vi "Write Data.vi"(8 "error in":errorcluster, 10 "Data":u16, 11 "U16 in":refnum<class "U16.lvclass">) -> (0 "error out":errorcluster, 3 "U16 out":refnum<class "U16.lvclass">)   [LabVIEW 2012, in "Base Data Class.lvlib" / "U16.lvclass"]
uses:
  U16.lvclass
  U16.lvclass/U16.ctl
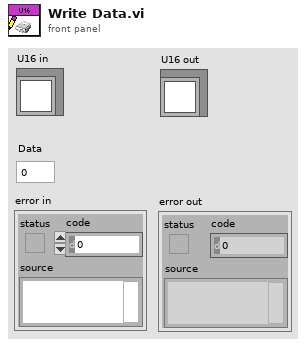
[diagram p1: front panel]
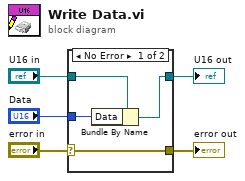
[diagram p0: block diagram]
diagram:
  n1 = case shown="No Error" "error in" {
    selector: "error in" -> [w9 w10]
    tunnel: [w9 w10] -> w4
    tunnel: [w7 w11] -> w2
    tunnel: "U16 in" -> [w8 w11]
    tunnel: "Data" -> [w6 _]
    frame No Error {
      n2 = Bundle By Name(cluster=w8, "Data"=w6) -> (w7:refnum<class "U16.lvclass">)
    }
    frame Error {
    }
  }
  "error out" <- w4
  "U16 out" <- w2
